vi "get_or_set_modifier_values.vi"(5 "modifier index":i32, 6 "clamp output values?":bool[](array[boolean]), 7 "action":T1, 8 "error in (no error)":errorcluster, 10 "modifier values in":dbl[](array[numeric]), 11 "GenericTrajectory in":refnum<class "TrajectoryDL121017Hopping.lvclass">) -> (0 "error out":errorcluster, 2 "modifier values out":dbl[](array[numeric]), 3 "GenericTrajectory out":refnum<class "TrajectoryDL121017Hopping.lvclass">)   [LabVIEW 2010, in "TrajectoryDL121017Hopping.lvclass"]
doc: "Gets, sets or resets the modifier values for all pixels of a trajectory. The first modifier (index = 0) typically belongs to a fast laser intensity modifier such as a Pockels cell.\n\nThe clamping values (one per pixel) indicate whether the modifier value for the corresponding pixels is clamped to zero (if true)."
uses:
  TrajectoryDL121017Hopping.lvclass
  common/enumerations/functional_global_action_enum.ctl
  TrajectoryDL091126GenericVoxel/TrajectoryDL091126GenericVoxel/TrajectoryDL091126GenericVoxel.lvclass
panel:
  out "clamping array size":i32
  out "clamping array":i16[](graph)
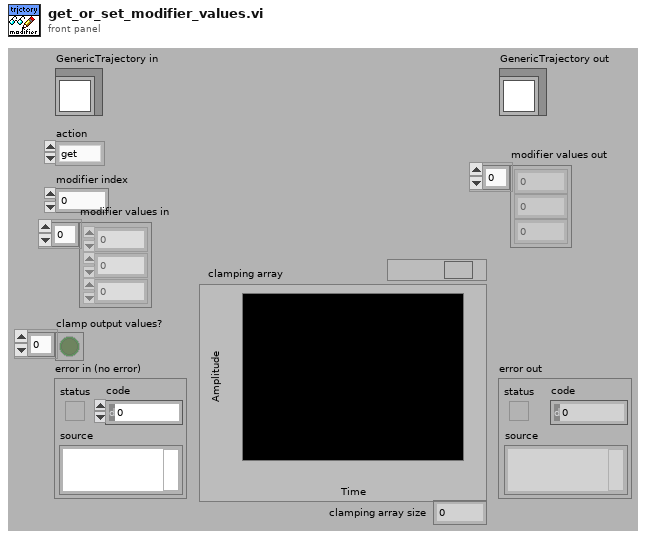
[diagram p1: front panel]
types:
  T1 = typedef "functional_global_action_enum.ctl" = enum16{"get", "set", "reset"}
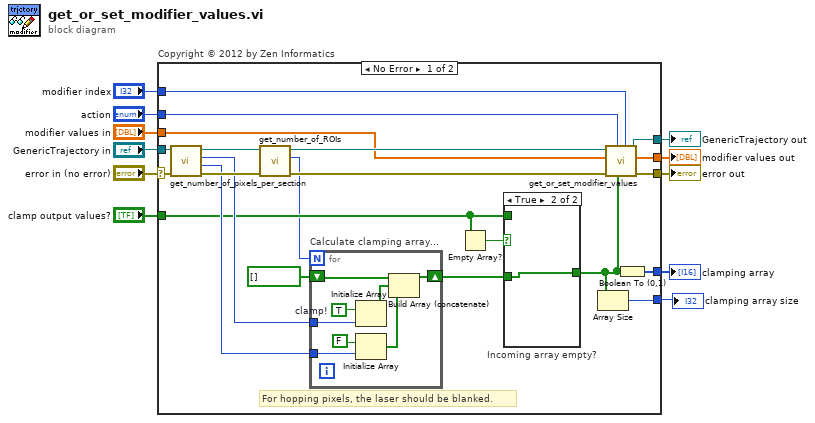
[diagram p0: block diagram]
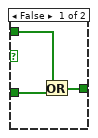
[diagram p2: hidden frame]
diagram:
  n1 = case "Copyright © 2012 by Zen Informatics" shown="No Error" "error in (no error)" {
    selector: "error in (no error)" -> [w28 w48]
    tunnel: [w33 w48] -> w11
    tunnel: [w32 w46] -> w10
    tunnel: [w31 w47] -> w9
    tunnel: "clamp output values?" -> [w20 _]
    tunnel: "modifier values in" -> [w16 w46]
    tunnel: "GenericTrajectory in" -> [w27 w47]
    tunnel: "modifier index" -> [w30 _]
    tunnel: "action" -> [w29 _]
    tunnel: [w18 _] -> w2
    tunnel: [w12 _] -> w1
    frame No Error {
      # "For hopping pixels, the laser should be blanked."
      n2 = call "get_number_of_pixels_per_section.vi"("error in (no error)"=w28, "TrajectoryDL121017Hopping in"=w27) -> ("error out"=w26:errorcluster, "pixels per uncaging section"=w21:i32, "pixels per hopping section"=w22:i32, "TrajectoryDL121017Hopping out"=w24:refnum<class "TrajectoryDL121017Hopping.lvclass">)  [unwired: 5 in, 1 out]
      n3 = call "get_number_of_ROIs.vi"("error in (no error)"=w26, "TrajectoryDL121017Hopping in"=w24) -> ("error out"=w25:errorcluster, "number of ROIs"=w17:i32, "TrajectoryDL121017Hopping out"=w23:refnum<class "TrajectoryDL121017Hopping.lvclass">)  [unwired: 7 in]
      n4 = for "Calculate clamping array..." {
        N: w17 -> [_]
        tunnel: w22 -> [w44]
        tunnel: w21 -> [w43]
        shift-right: [w38] -> w14
        shift-left: bool[] [] -> [w39]
        w45 = TRUE  # clamp!
        n5 = Initialize Array(w45, w44) -> (w41:bool[])
        n6 = Initialize Array(FALSE, w43) -> (w40:bool[])
        n7 = Build Array (concatenate)(w39, w41, w40) -> (w38:bool[])
      }
      n8 = Empty Array?(array=w20) -> (empty?=w19:bool)
      n9 = case "Incoming array empty?" shown="True" w19 {
        tunnel: [w36 w37] -> w13
        tunnel: w20 -> [w35 _]
        tunnel: w14 -> [w34 w37]
        frame False {
          n10 = Or(x=w35, y=w34) -> (x .or. y?=w36:bool[])
        }
        frame True {
        }
      }
      n11 = Array Size(array=w13) -> (size(s)=w12:i32)
      n12 = call-parent "get_or_set_modifier_values.vi"("modifier index"=w30, "clamp output values?"=w13, "action"=w29, "error in (no error)"=w25, "modifier values in"=w16, "GenericTrajectory in"=w23) -> ("error out"=w33:errorcluster, "modifier values out"=w32:dbl[], "GenericTrajectory out"=w31:refnum<class "TrajectoryDL121017Hopping.lvclass">)  [unwired: 3 in]
      n13 = Boolean To (0,1)(Boolean=w13) -> (0, 1=w18:i16[])
    }
    frame Error {
    }
  }
  "error out" <- w11
  "GenericTrajectory out" <- w9
  "modifier values out" <- w10
  "clamping array" <- w2
  "clamping array size" <- w1
